vi "Pre Launch Init.vi"(11 "Create Project View in":refnum<class "Edit Project View.lvclass">) -> (0 "error out":errorcluster, 3 "Create Project View out":refnum<class "Edit Project View.lvclass">)   [LabVIEW 2013, in "Edit Project View.lvlib" / "Edit Project View.lvclass"]
doc: "(<B>Filename</B>: Actor Framework.lvlib:Actor.lvclass:Pre Launch Init.vi)\n\nDefines behavior that occurs after the Launch Actor method is invoked but before the actor's Actor Core method begins running.\n\nThe Pre Launch Init method is guaranteed to finish before the Launch Actor method returns to its caller and before the actor itself receives any messages. Any references that the Pre Launch Init method obtains are guaranteed to have the same lifetime as the actor itself. Any errors that the Pre Launch Init method returns will abort the launch.\n\nBy default, this method does nothing. A descendant class may override it to define behavior."
uses:
  Edit Project View.lvclass
  Edit Project View.lvclass/Edit Project View.ctl
  <vilib>/ActorFrameworkMVC/View Actor/View Actor.lvclass
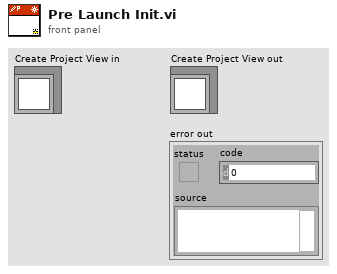
[diagram p1: front panel]
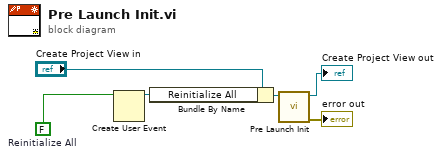
[diagram p0: block diagram]
diagram:
  w1 = FALSE  # Reinitialize All
  n1 = Create User Event(user event datatype=w1) -> (user event=w2:refnum<user-event>)  [unwired: 1 in, 1 out]
  n2 = Bundle By Name(cluster="Create Project View in", "Reinitialize All"=w2) -> (w3:refnum<class "Edit Project View.lvclass">)
  n3 = call-parent "Pre Launch Init.vi"("Actor in"=w3) -> ("error out"=→"error out":errorcluster, "Actor out"=→"Create Project View out":refnum<class "Edit Project View.lvclass">)  [unwired: 9 in]
